vi "Operate.vi"(0 "Divide in":refnum<class "Divide.lvclass">, 11 "error in (no error)":errorcluster) -> (4 "Divide out":refnum<class "Divide.lvclass">, 15 "error out":errorcluster)   [LabVIEW 2020, in "Divide.lvclass"]
uses:
  Divide.lvclass
  C:/Users/khishore.kumar/Khishore/labview_tips_2024/src/Assignment 25/Arithmetic Operations/Arithmetic Operations.lvclass
  Arithmetic Operations.lvclass/Arithmetic Operations.ctl
  Accessors/Read/Read A.vi
  Accessors/Read/Read B.vi
  Accessors/Write/Write C.vi
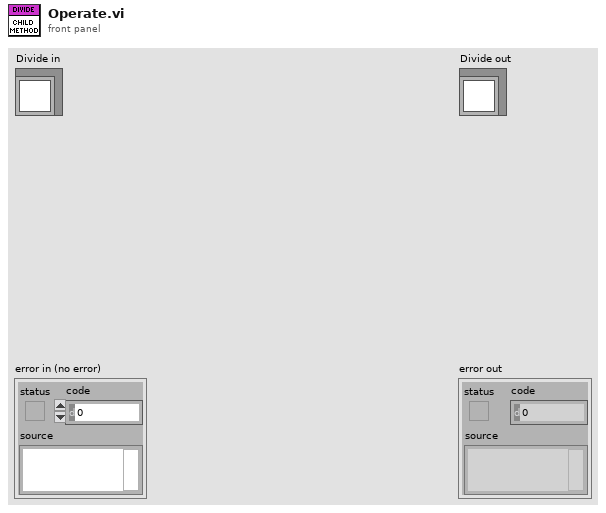
[diagram p1: front panel]
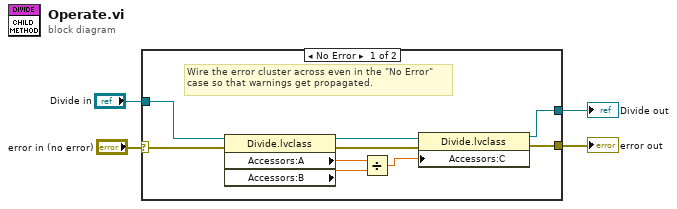
[diagram p0: block diagram]
diagram:
  n1 = case shown="No Error" "error in (no error)" {
    selector: "error in (no error)" -> [w13 w15]
    tunnel: [w11 w15] -> w3
    tunnel: [w6 w14] -> w1
    tunnel: "Divide in" -> [w10 w14]
    frame No Error {
      # "Wire the error cluster across even in the \"No Error\"\ncase so that warnings get propagated."
      n2 = property class="Divide.lvclass"(reference=w10, error in=w13) -> (reference out=w7:refnum<class "Divide.lvclass">, error out=w12:errorcluster, "Accessors:A"=w9:dbl, "Accessors:B"=w8:dbl)
      n3 = Divide(x=w9, y=w8) -> (x/y=w5:dbl)
      n4 = property class="Divide.lvclass"(reference=w7, error in=w12, "Accessors:C"=w5) -> (reference out=w6:refnum<class "Divide.lvclass">, error out=w11:errorcluster)
    }
    frame Error {
    }
  }
  "error out" <- w3
  "Divide out" <- w1
